vi "create data and colums (子VI).vi"(10 "结束时间":timestamp, 11 "seconds since 1Jan1904":timestamp) -> (2 "ColumnSetup":T2(array[cluster]), 3 "DataSource Data":string[][](array[string]))   [LabVIEW 2016]
uses:
  <vilib>/DataGrid for LabVIEW/source/GridColumn/ColumnType.ctl
  <vilib>/DataGrid for LabVIEW/source/GridColumn/GridColumn.lvclass
panel:
  out "lasttime":string
  out "foretime":string
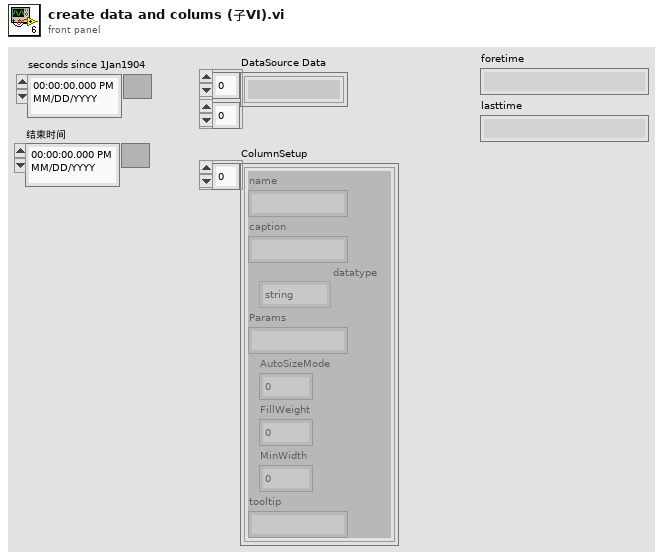
[diagram p1: front panel]
types:
  T1 = typedef "DataGrid.lvlib/GridColumn.lvclass/ColumnType.ctl" = enum16{"string", "image", "check", "numeric", "timestamp", "button", "combo", "link"}
  T2 = cluster{"name":string, "caption":string, "datatype":T1, "Params":string, "AutoSizeMode":i32, "FillWeight":sgl, "MinWidth":u32, "tooltip":string}[]
  T3 = cluster{"name":string, "caption":string, "datatype":T1, "Params":string, "AutoSizeMode":i32, "FillWeight":i32, "MinWidth":u32, "tooltip":string}
  T4 = typedef "NI_Database_API.lvlib/DB Tools DataTypes.ctl" = enum16{"String", "Long (I32)", "Single (SGL)", "Double (DBL)", "Date/Time", "Binary"}
  T5 = cluster{"name":string, "database data type":T4, "defined size":i32}[]
  T6 = cluster{"name":string, "caption":string, "datatype":T1, "Params":string, "AutoSizeMode":i32, "FillWeight":sgl, "MinWidth":u32, "tooltip":string}
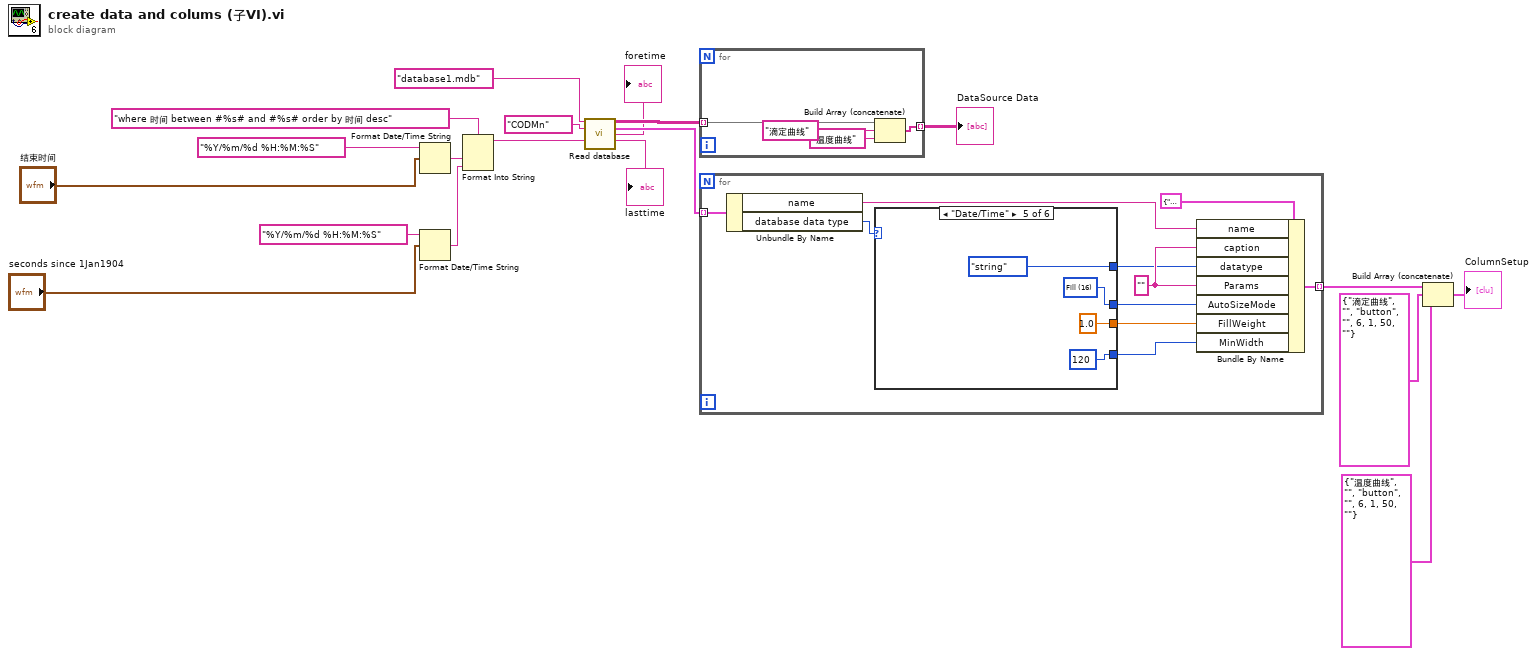
[diagram p0: block diagram]
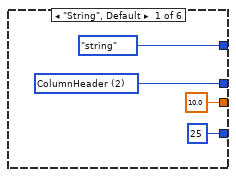
[diagram p2: hidden frame]
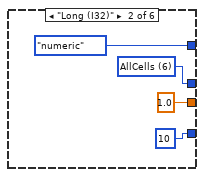
[diagram p3: hidden frame]
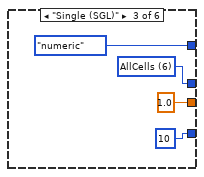
[diagram p4: hidden frame]
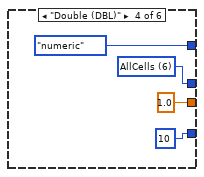
[diagram p5: hidden frame]
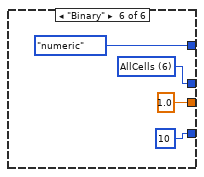
[diagram p6: hidden frame]
diagram:
  n1 = Format Date/Time String(time format string (%c)="%Y/%m/%d %H:%M:%S" ("时间格式字符串(%c)"), seconds (now)="结束时间") -> (date/time string=w15:string)  [unwired: 1 in]
  n2 = Format Date/Time String(time format string (%c)="%Y/%m/%d %H:%M:%S" ("时间格式字符串(%c)"), seconds (now)="seconds since 1Jan1904") -> (date/time string=w16:string)  [unwired: 1 in]
  n3 = Format Into String(format string="where 时间 between #%s# and #%s# order by 时间 desc" ("condition"), w15, w16) -> (resulting string=w17:string)  [unwired: 2 in, 1 out]
  n4 = call "Read database.vi"("database"="database1.mdb", "组合框"="CODMn", "condition"=w17) -> ("表格"=w10:string[][], "column information"=w6:T5, "foretime"=→"foretime":string, "lasttime"=→"lasttime":string)  [unwired: 7 in, 2 out]
  n5 = for {
    tunnel: w10 -> [w23] mode=indexing
    tunnel: [w21] -> w11 mode=indexing
    n6 = Build Array (concatenate)(w23, "滴定曲线" ("database"), "温度曲线" ("元素")) -> (w21:string[])
  }
  "DataSource Data" <- w11
  n7 = for {
    tunnel: w6 -> [w33] mode=indexing
    tunnel: [w30] -> w7 mode=indexing
    w28 = "" ("caption")
    n8 = Unbundle By Name(w33) -> ("name"=w29:string, "database data type"=w32:T4)
    n9 = case shown="\"Date/Time\"" w32 {
      tunnel: [ColumnType."string" ("datatype") ColumnType."numeric" ("datatype") ColumnType."numeric" ("datatype") ColumnType."numeric" ("datatype") ColumnType."string" ("datatype") ColumnType."numeric" ("datatype")] -> w27
      tunnel: [w36 w40 w45 w48 w52 w56] -> w26
      tunnel: [sgl 10.0 ("FillWeight") sgl 1.0 ("FillWeight") sgl 1.0 ("FillWeight") sgl 1.0 ("FillWeight") sgl 1.0 ("FillWeight") sgl 1.0 ("FillWeight")] -> w25
      tunnel: [u32 25 ("MinWidth") u32 10 ("MinWidth") u32 10 ("MinWidth") u32 10 ("MinWidth") u32 120 ("MinWidth") u32 10 ("MinWidth")] -> w24
      frame "String", Default {
        w36 = 2 items=["None"=1, "ColumnHeader"=2, "AllCellsExceptHeader"=4, "AllCells"=6, "DisplayedCellsExceptHeader"=8, "DisplayedCells"=10, "Fill"=16] ("AutoSizeMode")
      }
      frame "Long (I32)" {
        w40 = 6 items=["None"=1, "ColumnHeader"=2, "AllCellsExceptHeader"=4, "AllCells"=6, "DisplayedCellsExceptHeader"=8, "DisplayedCells"=10, "Fill"=16] ("AutoSizeMode")
      }
      frame "Single (SGL)" {
        w45 = 6 items=["None"=1, "ColumnHeader"=2, "AllCellsExceptHeader"=4, "AllCells"=6, "DisplayedCellsExceptHeader"=8, "DisplayedCells"=10, "Fill"=16] ("AutoSizeMode")
      }
      frame "Double (DBL)" {
        w48 = 6 items=["None"=1, "ColumnHeader"=2, "AllCellsExceptHeader"=4, "AllCells"=6, "DisplayedCellsExceptHeader"=8, "DisplayedCells"=10, "Fill"=16] ("AutoSizeMode")
      }
      frame "Date/Time" {
        w52 = 16 items=["None"=1, "ColumnHeader"=2, "AllCellsExceptHeader"=4, "AllCells"=6, "DisplayedCellsExceptHeader"=8, "DisplayedCells"=10, "Fill"=16] ("AutoSizeMode")
      }
      frame "Binary" {
        w56 = 6 items=["None"=1, "ColumnHeader"=2, "AllCellsExceptHeader"=4, "AllCells"=6, "DisplayedCellsExceptHeader"=8, "DisplayedCells"=10, "Fill"=16] ("AutoSizeMode")
      }
    }
    n10 = Bundle By Name(cluster=T6 {"name"="", "caption"="", "datatype"=enum."string", "Params"="", "AutoSizeMode"=1, "FillWeight"=100.0, "MinWidth"=50, "tooltip"=""}, "name"=w29, "caption"=w28, "datatype"=w27, "Params"=w28, "AutoSizeMode"=w26, "FillWeight"=w25, "MinWidth"=w24) -> (w30:T6)
  }
  n11 = Build Array (concatenate)(w7, T3 {"name"="滴定曲线", "caption"="", "datatype"=enum."button", "Params"="", "AutoSizeMode"=6, "FillWeight"=1, "MinWidth"=50, "tooltip"=""}, T3 {"name"="温度曲线", "caption"="", "datatype"=enum."button", "Params"="", "AutoSizeMode"=6, "FillWeight"=1, "MinWidth"=50, "tooltip"=""}) -> (→"ColumnSetup":T2)
